vi "Periodic Tasks.vi"(8 "error in":errorcluster) -> ()   [LabVIEW 2014]
doc: "This VI runs in parallel to other tasks. It can contain as many user-defined periodic loops as you need. These can carry out PID or other sorts of timed response."
uses:
  <vilib>/Rock Robotics/WPI/Joystick/WPI_JoystickGetSetRefNum.vi
  <vilib>/Rock Robotics/WPI/RobotDrive/WPI_RobotDriveGetSetRefNum.vi
  Robot Global Data.vi
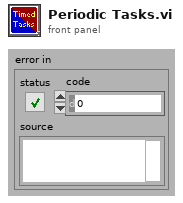
[diagram p1: front panel]
types:
  T1 = typedef "WPI_JoystickDevRef.ctl" = cluster{"Device":T2}
  T2 = typedef "WPI_JoystickDeviceEnum.ctl" = enum16{"USB 0", "USB 1", "USB 2", "USB 3", "USB 4", "USB 5"}
  T3 = typedef "WPI_RobotDriveDevRef.ctl" = cluster{"DevStatus":errorcluster, "Motors[]":T4[], "Square Inputs":bool, "Max Output":dbl}
  T4 = typedef "WPI_MotorControlDeviceRef.ctl" = cluster{"DeviceStatus":errorcluster, "Type":T5, "PWM":cluster{"Controller":T6, "PWM Channel":T7, "DeadBand":T8}, "CAN":cluster{"Device Number":u8, "Control Mode":T9, "Semaphore":T10, "Max Vout":dbl, "TalonSRX Control Mode":T11}, "Invert":bool, "TransformRef":T12, "InvTransformRef":T12}
  T5 = typedef "WPI_MotorControlType.ctl" = enum16{"PWM", "CAN", "CANTalonSRX"}
  T6 = typedef "FPGA_TypedefDigitalModule.ctl" = enum16{"Controller 1"}
  T7 = typedef "FPGA_DIOPWMChannel.ctl" = enum8{"PWM 0", "PWM 1", "PWM 2", "PWM 3", "PWM 4", "PWM 5", "PWM 6", "PWM 7", "PWM 8", "PWM 9", "PWM MXP 0", "PWM MXP 1", "PWM MXP 2", "PWM MXP 3", "PWM MXP 4", "PWM MXP 5", "PWM MXP 6", "PWM MXP 7", "PWM MXP 8", "PWM MXP 9", "Invalid"}
  T8 = typedef "WPI_PWMDeadband.ctl" = cluster{"Name":string, "maxPositivePwm":i32, "minPositivePwm":i32, "centerPwm":i32, "maxNegativePwm":i32, "minNegativePwm":i32, "angularRange":u16}
  T9 = typedef "WPI_CANJaguar_ControlMode.ctl" = enum8{"Percent VBus", "Current", "Speed", "Position", "Voltage"}
  T10 = typedef "Semaphore RefNum" = refnum<k1>
  T11 = typedef "WPI_CANTalonSRX_APIControlMode.ctl" = enum8{"Percent VBus", "Speed", "Position", "Slave", "Unchanged / Invalid"}
  T12 = typedef "WPI_PWMTransform_ConPane.ctl" = refnum<vi>
  T13 = cluster{"JoystickDevRef":T1, "RobotDriveDevRef":T3}
  T14 = typedef "WPI_DigitalInputDevRef.ctl" = cluster{"DevStatus":errorcluster, "DIO Channel":T15, "Controller":T6}
  T15 = typedef "FPGA_DIOChannel.ctl" = enum8{"DIO 0", "DIO 1", "DIO 2", "DIO 3", "DIO 4", "DIO 5", "DIO 6", "DIO 7", "DIO 8", "DIO 9", "DIO MXP 0", "DIO MXP 1", "DIO MXP 2", "DIO MXP 3", "DIO MXP 4", "DIO MXP 5", "DIO MXP 6", "DIO MXP 7", "DIO MXP 8", "DIO MXP 9", "DIO MXP 10", "DIO MXP 11", "DIO MXP 12", "DIO MXP 13", "DIO MXP 14", "DIO MXP 15", "Invalid"}
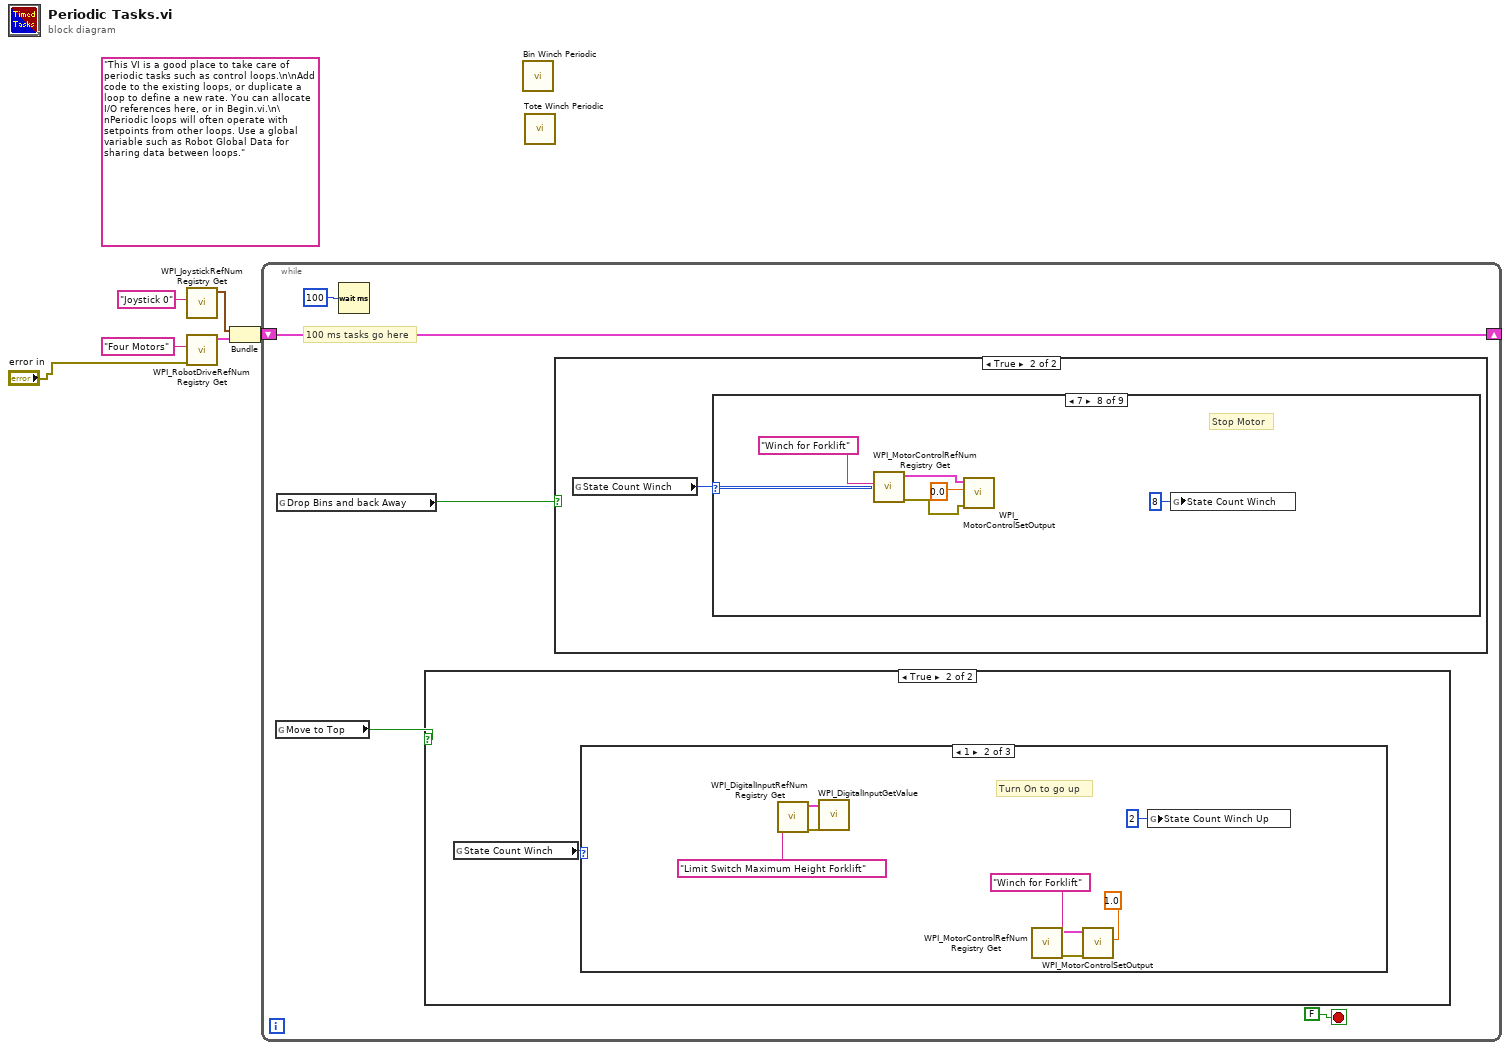
[diagram p0: block diagram]
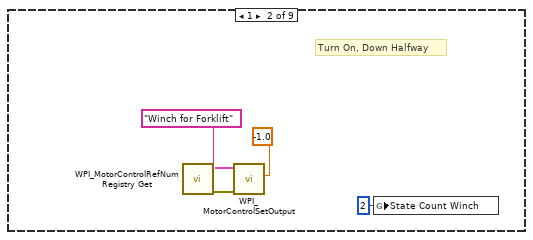
[diagram p7: hidden frame]
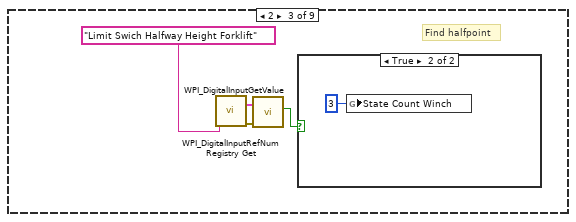
[diagram p8: hidden frame]
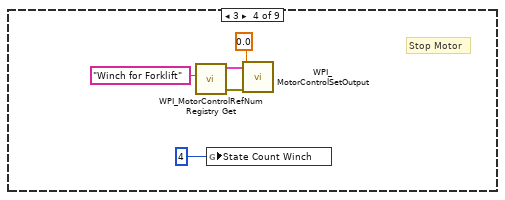
[diagram p10: hidden frame]
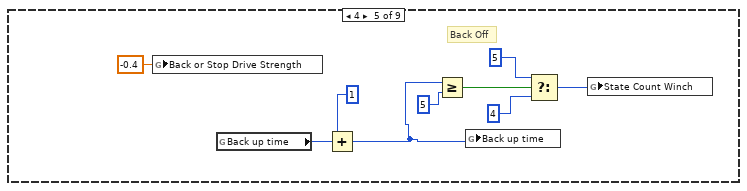
[diagram p11: hidden frame]
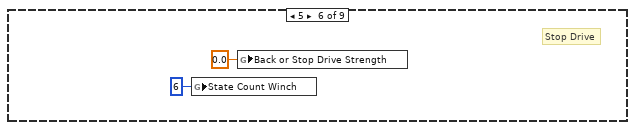
[diagram p12: hidden frame]
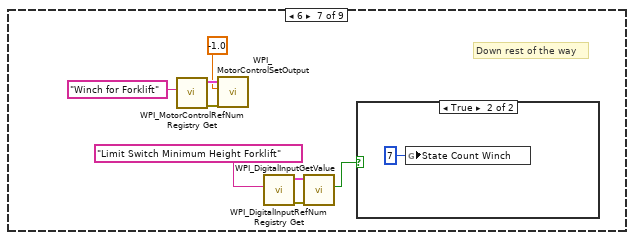
[diagram p13: hidden frame]
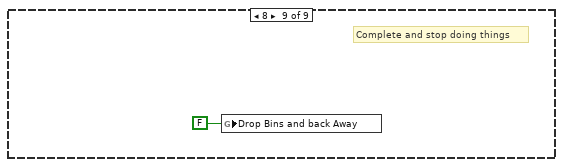
[diagram p15: hidden frame]
diagram:
  (unwired) "This VI is a good place to take care of periodic tasks such as control loops.\n\nAdd code to the existing loops, or duplicate a loop to define a new rate. You can allocate I/O references here, or in Begin.vi.\n\nPeriodic loops will often operate with setpoints from other loops. Use a global variable such as Robot Global Data for sharing data between loops."
  n1 = call <vilib>:"WPI_JoystickRefNum Registry Get.vi"("refnum name"="Joystick 0") -> ("JoystickDevRef"=w4:T1)  [unwired: 1 in, 9 out]
  n2 = call <vilib>:"WPI_RobotDriveRefNum Registry Get.vi"("error in (no error)"="error in", "refnum name"="Four Motors") -> ("RobotDriveDevRef"=w3:T3)  [unwired: 9 out]
  n3 = Bundle("JoystickDevRef"=w4, "RobotDriveDevRef"=w3) -> (w2:T13)  [unwired: 1 out]
  n4 = while {
    shift-right: [w9] -> _
    shift-left: w2 -> [w9]
    stop <- FALSE stop-if-true
    # "100 ms tasks go here"
    n5 = global read "Robot Global Data.vi" "Move to Top"() -> (w7:bool)
    n6 = global read "Robot Global Data.vi" "Drop Bins and back Away"() -> (w8:bool)
    n7 = Wait (ms)(milliseconds to wait=u32 100) -> ()  [unwired: 1 out]
    n8 = case shown="True" w7 {
      frame False {
      }
      frame True {
        n9 = global read "Robot Global Data.vi" "State Count Winch"() -> (w12:i16)
        n10 = case shown="1" w12 {
          frame 0, Default {
            # "Do Nothing"
          }
          frame 1 {
            # "Turn On to go up"
            n11 = call <vilib>:"WPI_DigitalInputRefNum Registry Get.vi"("refnum name"="Limit Switch Maximum Height Forklift") -> ("error out"=w15:errorcluster, "DigitalInputDevRef"=w14:T14)  [unwired: 9 in]
            n12 = call <vilib>:"WPI_DigitalInputGetValue.vi"("error in (no error)"=w15, "DigitalInputDevRef"=w14) -> ()  [unwired: 7 in, 3 out]
            n13 = call <vilib>:"WPI_MotorControlRefNum Registry Get.vi"("refnum name"="Winch for Forklift") -> ("error out"=w17:errorcluster, "MotorControlDevRef"=w18:T4)  [unwired: 9 in]
            n14 = call <vilib>:"WPI_MotorControlSetOutput.vi"("error in (no error)"=w17, "Output"=1.0, "MotorControlDevRef"=w18) -> ()  [unwired: 6 in, 3 out]
            n15 = global write "Robot Global Data.vi" "State Count Winch Up"(i16 2 ("State Count Winch Up")) -> ()
          }
          frame 2 {
            # "Stop at top"
          }
        }
      }
    }
    n16 = case shown="True" w8 {
      frame False {
      }
      frame True {
        n17 = global read "Robot Global Data.vi" "State Count Winch"() -> (w21:i16)
        n18 = case shown="7" w21 {
          frame 0, Default {
            # "Do Nothing"
          }
          frame 1 {
            # "Turn On, Down Halfway"
            n19 = call <vilib>:"WPI_MotorControlRefNum Registry Get.vi"("refnum name"="Winch for Forklift") -> ("error out"=w23:errorcluster, "MotorControlDevRef"=w24:T4)  [unwired: 9 in]
            n20 = call <vilib>:"WPI_MotorControlSetOutput.vi"("error in (no error)"=w23, "Output"=-1.0, "MotorControlDevRef"=w24) -> ()  [unwired: 6 in, 3 out]
            n21 = global write "Robot Global Data.vi" "State Count Winch"(i16 2 ("State Count Winch")) -> ()
          }
          frame 2 {
            # "Find halfpoint"
            n22 = call <vilib>:"WPI_DigitalInputRefNum Registry Get.vi"("refnum name"="Limit Swich Halfway Height Forklift") -> ("error out"=w30:errorcluster, "DigitalInputDevRef"=w29:T14)  [unwired: 9 in]
            n23 = call <vilib>:"WPI_DigitalInputGetValue.vi"("error in (no error)"=w30, "DigitalInputDevRef"=w29) -> ("Value"=w27:bool)  [unwired: 7 in, 2 out]
            n24 = case shown="True" w27 {
              frame False {
              }
              frame True {
                n25 = global write "Robot Global Data.vi" "State Count Winch"(i16 3 ("State Count Winch")) -> ()
              }
            }
          }
          frame 3 {
            # "Stop Motor"
            n26 = call <vilib>:"WPI_MotorControlRefNum Registry Get.vi"("refnum name"="Winch for Forklift") -> ("error out"=w36:errorcluster, "MotorControlDevRef"=w35:T4)  [unwired: 9 in]
            n27 = global write "Robot Global Data.vi" "State Count Winch"(i16 4 ("State Count Winch")) -> ()
            n28 = call <vilib>:"WPI_MotorControlSetOutput.vi"("error in (no error)"=w36, "Output"=0.0, "MotorControlDevRef"=w35) -> ()  [unwired: 6 in, 3 out]
          }
          frame 4 {
            # "Back Off"
            n29 = global write "Robot Global Data.vi" "Back or Stop Drive Strength"(-0.4 ("Back or Stop Drive Strength")) -> ()
            n30 = global read "Robot Global Data.vi" "Back up time"() -> (w45:i16)
            n31 = Add(x=i16 1, y=w45) -> (x+y=w43:i16)
            n32 = Greater Or Equal?(x=w43, y=i16 5) -> (x >= y?=w41:bool)
            n33 = global write "Robot Global Data.vi" "Back up time"(w43) -> ()
            n34 = Select(t=i16 5, s=w41, f=i16 4) -> (s? t:f=w40:i16)
            n35 = global write "Robot Global Data.vi" "State Count Winch"(w40) -> ()
          }
          frame 5 {
            # "Stop Drive"
            n36 = global write "Robot Global Data.vi" "State Count Winch"(i16 6 ("State Count Winch")) -> ()
            n37 = global write "Robot Global Data.vi" "Back or Stop Drive Strength"(0.0 ("Back or Stop Drive Strength")) -> ()
          }
          frame 6 {
            # "Down rest of the way"
            n38 = call <vilib>:"WPI_MotorControlRefNum Registry Get.vi"("refnum name"="Winch for Forklift") -> ("error out"=w55:errorcluster, "MotorControlDevRef"=w54:T4)  [unwired: 9 in]
            n39 = call <vilib>:"WPI_MotorControlSetOutput.vi"("error in (no error)"=w55, "Output"=-1.0 ("Motor Output"), "MotorControlDevRef"=w54) -> ()  [unwired: 6 in, 3 out]
            n40 = call <vilib>:"WPI_DigitalInputRefNum Registry Get.vi"("refnum name"="Limit Switch Minimum Height Forklift") -> ("error out"=w51:errorcluster, "DigitalInputDevRef"=w50:T14)  [unwired: 9 in]
            n41 = call <vilib>:"WPI_DigitalInputGetValue.vi"("error in (no error)"=w51, "DigitalInputDevRef"=w50) -> ("Value"=w48:bool)  [unwired: 7 in, 2 out]
            n42 = case shown="True" w48 {
              frame False {
              }
              frame True {
                n43 = global write "Robot Global Data.vi" "State Count Winch"(i16 7 ("State Count Winch")) -> ()
              }
            }
          }
          frame 7 {
            # "Stop Motor"
            n44 = call <vilib>:"WPI_MotorControlRefNum Registry Get.vi"("refnum name"="Winch for Forklift") -> ("error out"=w57:errorcluster, "MotorControlDevRef"=w58:T4)  [unwired: 9 in]
            n45 = call <vilib>:"WPI_MotorControlSetOutput.vi"("error in (no error)"=w57, "Output"=0.0 ("Motor Output"), "MotorControlDevRef"=w58) -> ()  [unwired: 6 in, 3 out]
            n46 = global write "Robot Global Data.vi" "State Count Winch"(i16 8 ("State Count Winch")) -> ()
          }
          frame 8 {
            # "Complete and stop doing things"
            n47 = global write "Robot Global Data.vi" "Drop Bins and back Away"(FALSE) -> ()
          }
        }
      }
    }
  }
  n48 = call "Bin Winch Periodic.vi"() -> ()  [unwired: 12 in]
  n49 = call "Tote Winch Periodic.vi"() -> ()  [unwired: 12 in]
